vi "ToRepo.vi"(8 "error in":errorcluster, 9 "to repo cluster":T1, 10 "repository in":refnum<class "NISE_CEF_Repository.lvclass">, 11 "node in":refnum<class "Targets.lvclass">) -> (0 "error out":errorcluster, 2 "repository out":refnum<class "NISE_CEF_Repository.lvclass">, 3 "node out":refnum<class "Targets.lvclass">)   [LabVIEW 2015, in "Targets.lvclass"]
doc: "Transfers the information from the tree node into the repo. How it is stored in the repo depends on the Repo.Copyright 2015 National Instruments Corporation\n\nLicensed under the Apache License, Version 2.0 (the \"License\"); you may not use this file except in compliance with the License. You may obtain a copy of the License at http://www.apache.org/licenses/LICENSE-2.0\nUnless required by applicable law or agreed to in writing, software distributed under the License is distributed on an \"AS IS\" BASIS, WITHOUT WARRANTIES OR CONDITIONS OF ANY KIND, either express or implied. See the License for the specific language governing permissions and limitations under the License."
uses:
  Targets.lvclass
  <vilib>/NI/Configuration Framework/Repository/NISE_CEF_Repository.lvclass
  <vilib>/NI/Configuration Framework/Node/ToRepoCluster.ctl
  CustomDeviceRepo/CustomDeviceRepo.lvclass
  <vilib>/NI/Configuration Framework/Node/NISE_CEF_Node.lvclass/NISE_CEF_Node.ctl
  Target/Target.lvclass
  Target/Target.lvclass/Target.ctl
  CustomDeviceRepo/CustomDeviceRepo.lvclass/CustomDeviceRepo.ctl
  Target/Read Source.vi
  <vilib>/NI/Configuration Framework/Node/ReadChildren.vi
  CustomDeviceRepo/Write Supported Targets Properties.vi
  <vilib>/NI/Configuration Framework/Node/NISE_CEF_Node.lvclass
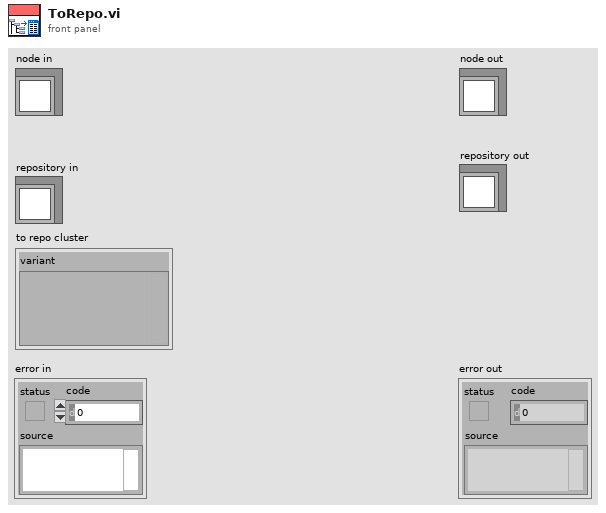
[diagram p1: front panel]
types:
  T1 = typedef "NISE_CEF_Node.lvclass/ToRepoCluster.ctl" = cluster{"variant":variant}
  T2 = typedef "NISE_CEF_Node.lvclass/NodeRef.ctl" = refnum<data-value>
  T3 = typedef "Configuration Tool.lvlib/Path Cluster.ctl" = cluster{"Path":path, "Path Type":enum16{"Absolute", "To Base", "To Common Doc Dir", "To Application Data Dir"}}
  T4 = typedef "Configuration Tool.lvlib/Target.ctl" = enum16{"All", "Pharlap", "VxWorks", "Windows", "Linux_32_ARM", "Linux_x64", "PharlapWindows", "PharlapVxWorks", "VxWorksWindows"}
  T5 = cluster{"Source":T3, "Real Time System Destination":string, "Supported Target":T4}
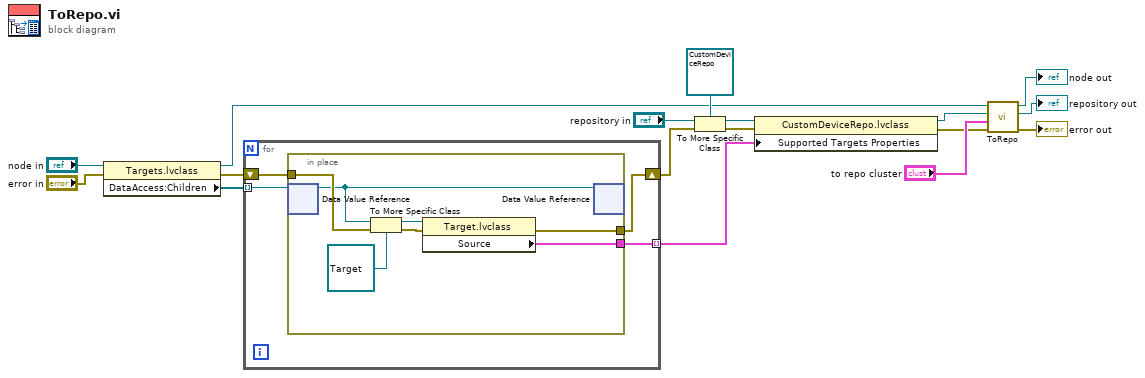
[diagram p0: block diagram]
diagram:
  n1 = property class="Targets.lvclass"(reference="node in", error in="error in") -> (reference out=w1:refnum<class "Targets.lvclass">, error out=w8:errorcluster, "DataAccess:Children"=w7:T2[])
  n2 = for {
    shift-right: [w19] -> w6
    shift-left: w8 -> [w20]
    tunnel: w7 -> [w21] mode=indexing
    tunnel: [w18] -> w5 mode=indexing
    n3 = in-place {
      in-place-border: w20 -> [w28]
      in-place-border: [w23] -> w18
      in-place-border: [w22] -> w19
      n4 = in-place-dvr #1(w21) -> (w26:refnum<class "NISE_CEF_Node.lvclass">)  [unwired: 1 out]
      n5 = To More Specific Class(target class=refnum<class "Target.lvclass"> refnum ("Target.lvclass"), reference=w26, error in=w28) -> (specific class reference=w25:refnum<class "Target.lvclass">, error out=w24:errorcluster)
      n6 = property class="Target.lvclass"(reference=w25, error in=w24) -> (error out=w22:errorcluster, "Source"=w23:T5)  [unwired: 1 out]
      n7 = in-place-dvr #1(w26) -> ()  [unwired: 2 out]
    }
  }
  n8 = To More Specific Class(target class=refnum<class "CustomDeviceRepo.lvclass"> refnum ("CustomDeviceRepo.lvclass"), reference="repository in", error in=w6) -> (specific class reference=w14:refnum<class "CustomDeviceRepo.lvclass">, error out=w13:errorcluster)
  n9 = property class="CustomDeviceRepo.lvclass"(reference=w14, error in=w13, "Supported Targets Properties"=w5) -> (reference out=w3:refnum<class "CustomDeviceRepo.lvclass">, error out=w4:errorcluster)
  n10 = call-parent "ToRepo.vi"("error in"=w4, "to repo cluster"="to repo cluster", "repository in"=w3, "node in"=w1) -> ("error out"=→"error out":errorcluster, "repository out"=→"repository out":refnum<class "NISE_CEF_Repository.lvclass">, "node out"=→"node out":refnum<class "Targets.lvclass">)  [unwired: 5 in]
